vi "update.links.vi"(8 "error in (no error)":errorcluster, 10 "Links":map{string, string}(c390), 11 "Run in":refnum<class "Run.lvclass">) -> (0 "error out":errorcluster, 3 "Run out":refnum<class "Run.lvclass">)   [LabVIEW 2020, in "Run.lvclass"]
uses:
  Run.lvclass
  Nominal Client/Nominal Client.lvclass
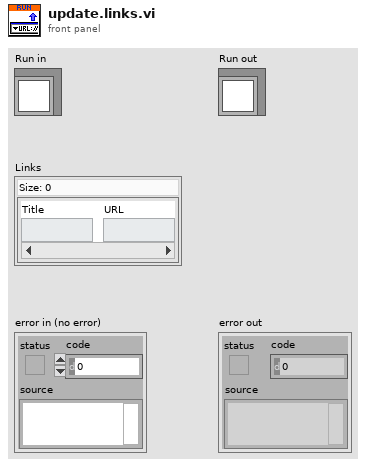
[diagram p1: front panel]
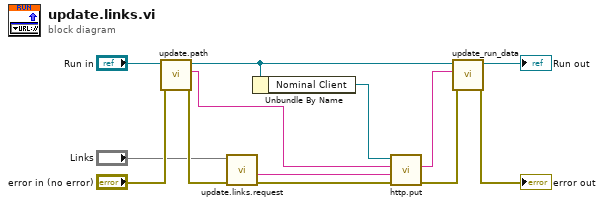
[diagram p0: block diagram]
diagram:
  n1 = call "update.path.vi"("error in"="error in (no error)", "Run"="Run in") -> ("error out"=w11:errorcluster, "path"=w8:string, "Run Out"=w5:refnum<class "Run.lvclass">)  [unwired: 7 in]
  n2 = call "update.links.request.vi"("error in"=w11, "Links"="Links") -> ("error out"=w6:errorcluster, "Request"=w7:string)  [unwired: 8 in]
  n3 = Unbundle By Name(w5) -> ("Nominal Client"=w9:refnum<class "Nominal Client.lvclass">)
  n4 = call "http.put.vi"("error in"=w6, "Body"=w7, "Path"=w8, "Nominal Client in"=w9) -> ("error out"=w3:errorcluster, "Response"=w4:string)  [unwired: 5 in, 1 out]
  n5 = call "update_run_data.vi"("error in"=w3, "Run JSON"=w4, "Run in"=w5) -> ("error out"=→"error out":errorcluster, "Run out"=→"Run out":refnum<class "Run.lvclass">)  [unwired: 7 in]
